vi "Update RPC Client Method Constants.vi"(5 "Library":refnum<vi>, 6 "RPC Method Parameters":T1, 8 "error in (no error)":errorcluster, 11 "VI in":refnum<vi>) -> (0 "error out":errorcluster, 3 "VI out":refnum<vi>)   [LabVIEW 2019, in "gRPC Template Creation Utility.lvlib"]
uses:
  gRPC Template Creation Utility.lvlib
  <vilib>/Utility/traverseref.llb/TRef TravTarget.ctl
  0eaa7444-8baf-4465-b530-593cae42fb70.vi
  <vilib>/Comparison/Equal/Equal Functor/Equal Functor.lvclass
  <vilib>/Utility/traverseref.llb/VI Scripting - Traverse.lvlib
  TypeDefs/RPC Method Parameters.ctl
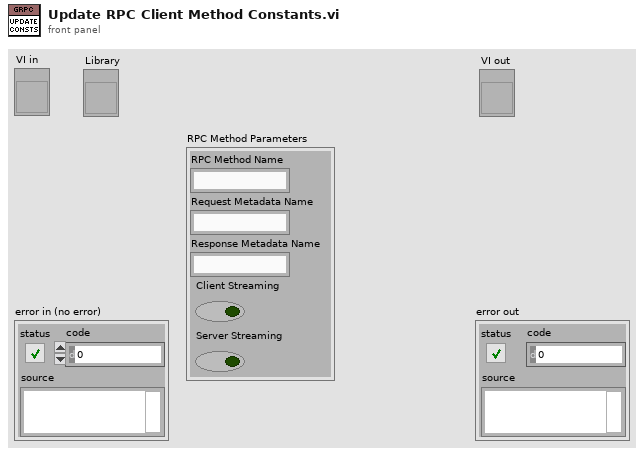
[diagram p1: front panel]
types:
  T1 = typedef "gRPC Template Creation Utility.lvlib/RPC Method Parameters.ctl" = cluster{"RPC Method Name":string, "Request Metadata Name":string, "Response Metadata Name":string, "Client Streaming":bool, "Server Streaming":bool}
  T2 = typedef "TRef TravTarget.ctl" = enum16{"FP", "BD", "Other"}
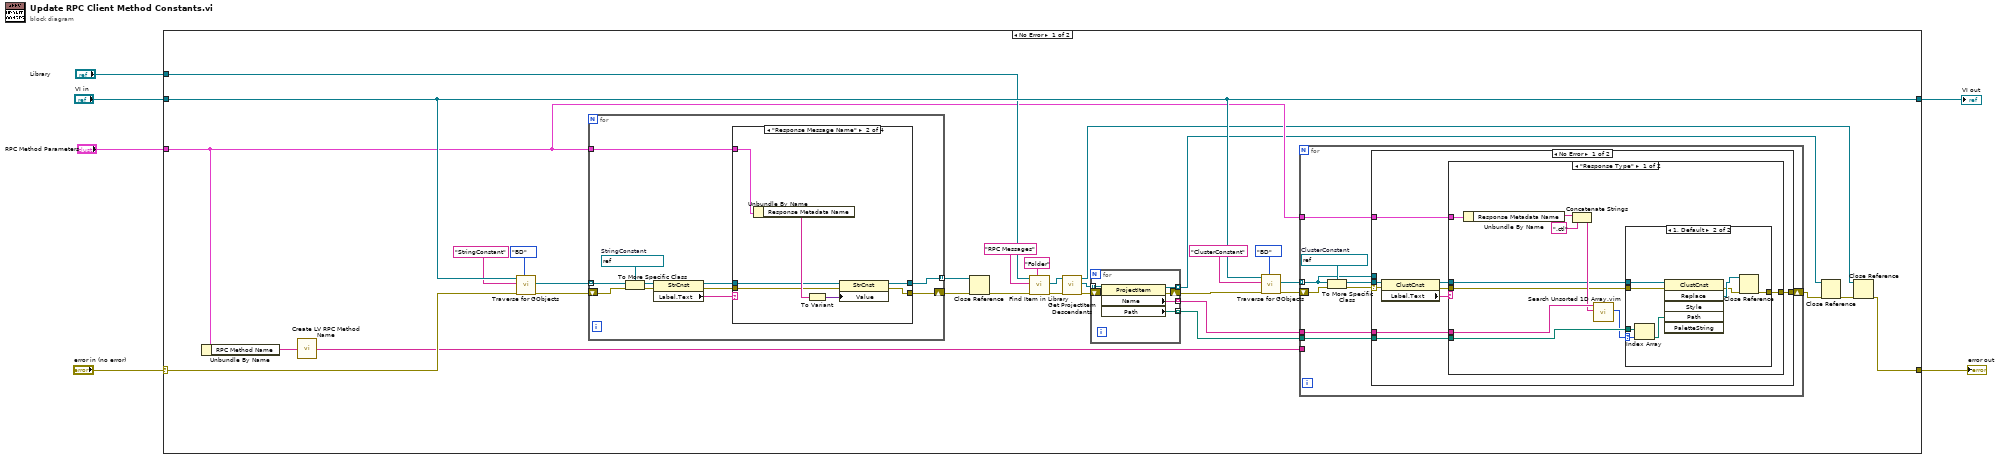
[diagram p0: block diagram]
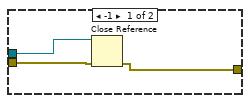
[diagram p2: hidden frame]
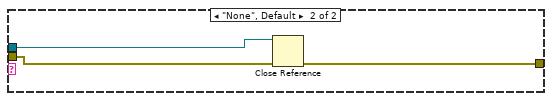
[diagram p3: hidden frame]
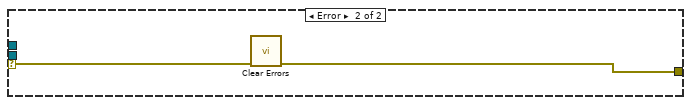
[diagram p4: hidden frame]
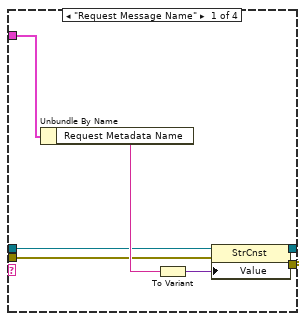
[diagram p5: hidden frame]
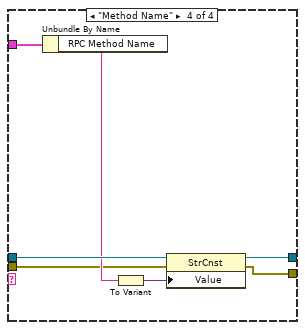
[diagram p7: hidden frame]
diagram:
  n1 = case shown="No Error" "error in (no error)" {
    selector: "error in (no error)" -> [w36 w123]
    tunnel: [w37 w123] -> w6
    tunnel: "VI in" -> [w35 w122]
    tunnel: [w35 w122] -> w3
    tunnel: "Library" -> [w34 _]
    tunnel: "RPC Method Parameters" -> [w33 _]
    frame No Error {
      n2 = Unbundle By Name(w33) -> ("RPC Method Name"=w32:string)
      n3 = call "Create LV RPC Method Name.vi"("Proto Parser RPC Method Name in"=w32) -> ("LV RPC Method Name out"=w31:string)
      n4 = call <vilib>:"Traverse for GObjects.vi"("Traverse Target"=TRef_TravTarget."BD", "error in (no error)"=w36, "Class Name"="StringConstant", "VI Refnum"=w35) -> ("error out"=w28:errorcluster, "References"=w24:refnum<vi>[])  [unwired: 4 in, 2 out]
      n5 = for {
        tunnel: w24 -> [w97] mode=indexing
        shift-right: [w89] -> w25
        shift-left: w28 -> [w96]
        tunnel: w33 -> [w92]
        tunnel: [w88] -> w23 mode=indexing
        w98 = refnum<vi> refnum  # StringConstant
        n6 = To More Specific Class(target class=w98, reference=w97, error in=w96) -> (specific class reference=w95:refnum<vi>, error out=w94:errorcluster)
        n7 = property class="StrCnst"(reference=w95, error in=w94) -> (reference out=w91:refnum<vi>, error out=w90:errorcluster, "Label.Text"=w93:string)
        n8 = case shown="\"Response Message Name\"" w93 {
          tunnel: w92 -> [w100 w110 _ w121]
          tunnel: w91 -> [w102 w108 w113 w120]
          tunnel: w90 -> [w103 w109 w114 w117]
          tunnel: [w101 w107 w114 w116] -> w89
          tunnel: [w99 w106 w113 w115] -> w88
          frame "Request Message Name" {
            n9 = Unbundle By Name(w100) -> ("Request Metadata Name"=w105:string)
            n10 = To Variant(anything=w105) -> (Variant=w104:variant)
            n11 = property class="StrCnst"(reference=w102, error in=w103, "Value"=w104) -> (reference out=w99:refnum<vi>, error out=w101:errorcluster)
          }
          frame "Response Message Name" {
            n12 = Unbundle By Name(w110) -> ("Response Metadata Name"=w112:string)
            n13 = To Variant(anything=w112) -> (Variant=w111:variant)
            n14 = property class="StrCnst"(reference=w108, error in=w109, "Value"=w111) -> (reference out=w106:refnum<vi>, error out=w107:errorcluster)
          }
          frame "None", Default {
          }
          frame "Method Name" {
            n15 = Unbundle By Name(w121) -> ("RPC Method Name"=w119:string)
            n16 = To Variant(anything=w119) -> (Variant=w118:variant)
            n17 = property class="StrCnst"(reference=w120, error in=w117, "Value"=w118) -> (reference out=w115:refnum<vi>, error out=w116:errorcluster)
          }
        }
      }
      n18 = Close Reference(reference=w23, error in (no error)=w25) -> (error out=w15:errorcluster)
      n19 = call "Find Item in Library.vi"("Item Type"="Folder", "error in (no error)"=w15, "Item Name"="RPC Messages", "Library item in"=w34) -> ("error out"=w19:errorcluster, "Project Item (Library Item)"=w18:refnum<vi>)  [unwired: 4 in, 2 out]
      n20 = call "Get ProjectItem Descendants.vi"("error in (no error)"=w19, "ProjectItem in"=w18) -> ("error out"=w14:errorcluster, "All Descendents"=w20:refnum<vi>[], "ProjectItem out"=w12:refnum<vi>)  [unwired: 7 in]
      n21 = for {
        tunnel: w20 -> [w43] mode=indexing
        tunnel: [w42] -> w10 mode=indexing
        tunnel: [w41] -> w9 mode=indexing
        shift-right: [w39] -> w13
        shift-left: w14 -> [w40]
        tunnel: [w38] -> w8 mode=indexing
        n22 = property class="ProjectItem"(reference=w43, error in=w40) -> (reference out=w41:refnum<vi>, error out=w39:errorcluster, "Name"=w42:string, "Path"=w38:path)
      }
      n23 = call <vilib>:"Traverse for GObjects.vi"("Traverse Target"=TRef_TravTarget."BD", "error in (no error)"=w13, "Class Name"="ClusterConstant", "VI Refnum"=w35) -> ("error out"=w22:errorcluster, "References"=w21:refnum<vi>[])  [unwired: 4 in, 2 out]
      n24 = for {
        tunnel: w21 -> [w44] mode=indexing
        shift-right: [w48] -> w11
        shift-left: w22 -> [w51]
        tunnel: w31 -> [_]
        tunnel: w33 -> [w47]
        tunnel: w10 -> [w46]
        tunnel: w8 -> [w45]
        w52 = refnum<vi> refnum  # ClusterConstant
        n25 = To More Specific Class(target class=w52, reference=w44, error in=w51) -> (specific class reference=w50:refnum<vi>, error out=w49:errorcluster)
        n26 = case shown="No Error" w49 {
          selector: w49 -> [w60 w87]
          tunnel: w50 -> [w61 _]
          tunnel: [w56 w86] -> w48
          tunnel: w47 -> [w55 _]
          tunnel: w46 -> [w54 _]
          tunnel: w45 -> [w53 _]
          tunnel: w44 -> [_ _]
          frame No Error {
            n27 = property class="ClustCnst"(reference=w61, error in=w60) -> (reference out=w58:refnum<vi>, error out=w57:errorcluster, "Label.Text"=w59:string)
            n28 = case shown="\"Response Type\"" w59 {
              tunnel: w58 -> [w64 w85]
              tunnel: w57 -> [w63 w84]
              tunnel: [w62 w83] -> w56
              tunnel: w55 -> [w71 _]
              tunnel: w54 -> [w68 _]
              tunnel: w53 -> [w66 _]
              frame "Response Type" {
                n29 = Unbundle By Name(w71) -> ("Response Metadata Name"=w70:string)
                n30 = Concatenate Strings(w70, ".ctl" ("string")) -> (w67:string)
                n31 = call "Search Unsorted 1D Array.vim"("element"=w67, "unsorted 1D array"=w68) -> ("index of element"=w65:i32)  [unwired: 9 in]
                n32 = case shown="1, Default" w65 {
                  selector: w65 -> [_ w81]
                  tunnel: w66 -> [_ w82]
                  tunnel: w64 -> [w74 w80]
                  tunnel: w63 -> [w73 w79]
                  tunnel: [w72 w75] -> w62
                  frame -1 {
                    n33 = Close Reference(reference=w74, error in (no error)=w73) -> (error out=w72:errorcluster)
                  }
                  frame 1, Default {
                    n34 = Index Array(array=w82, index=w81) -> (element=w78:path)
                    n35 = invoke class="ClustCnst" method="Replace"(reference=w80, error in=w79, "Path"=w78) -> (error out=w76:errorcluster, "Replace"=w77:refnum<vi>)  [unwired: 3 in, 4 out]
                    n36 = Close Reference(reference=w77, error in (no error)=w76) -> (error out=w75:errorcluster)
                  }
                }
              }
              frame "None", Default {
                n37 = Close Reference(reference=w85, error in (no error)=w84) -> (error out=w83:errorcluster)
              }
            }
          }
          frame Error {
            n38 = call <vilib>:"Clear Errors.vi"("error in (no error)"=w87) -> ("error out"=w86:errorcluster)  [unwired: 5 in, 1 out]
          }
        }
      }
      n39 = Close Reference(reference=w9, error in (no error)=w11) -> (error out=w7:errorcluster)
      n40 = Close Reference(reference=w12, error in (no error)=w7) -> (error out=w37:errorcluster)
    }
    frame Error {
    }
  }
  "error out" <- w6
  "VI out" <- w3
